vi "CommandZaber.vi"(0 "Zaber":T2={"Serial port handle"="", "Axis"="", "Controller #"=0, "Min position"=0.0, "Max position"=0.0, "Min velocity"=0.0, "Max velocity"=0.0, "Firmware"="", "Device ID"=0, "Variable event"=refnum, "Variable ref"=refnum, "Resolution, usteps/step"=0, "Serial port semaphore"=refnum, "Joystick buttons"={"MinDir"=1, "MaxDir"=2, "MedSpeed"=5, "HighSpeed"=6}} {"Joystick buttons"."HighSpeed" min=1 max=25 step=1; "Joystick buttons"."MedSpeed" min=1 max=25 step=1; "Joystick buttons"."MaxDir" min=1 max=25 step=1; "Joystick buttons"."MinDir" min=1 max=25 step=1}, 2 "Command":T1, 5 "error in":errorcluster) -> (11 "Command time, ms":u32, 14 "Zaber out":T2={"Serial port handle"="", "Axis"="", "Controller #"=0, "Min position"=0.0, "Max position"=0.0, "Min velocity"=0.0, "Max velocity"=0.0, "Firmware"="", "Device ID"=0, "Variable event"=refnum, "Variable ref"=refnum, "Resolution, usteps/step"=0, "Serial port semaphore"=refnum, "Joystick buttons"={"MinDir"=1, "MaxDir"=2, "MedSpeed"=5, "HighSpeed"=6}} {"Joystick buttons"."HighSpeed" min=1 max=25 step=1; "Joystick buttons"."MedSpeed" min=1 max=25 step=1; "Joystick buttons"."MaxDir" min=1 max=25 step=1; "Joystick buttons"."MinDir" min=1 max=25 step=1}, 16 "Answer":T1, 19 "error out":errorcluster)   [LabVIEW 2018]
uses:
  Zaber.ctl
  GenericDataEvent/GenericEvent.ctl
  ZaberVariables.ctl
  CommandZaber.ctl
panel:
  out "Bytes at Port":u32
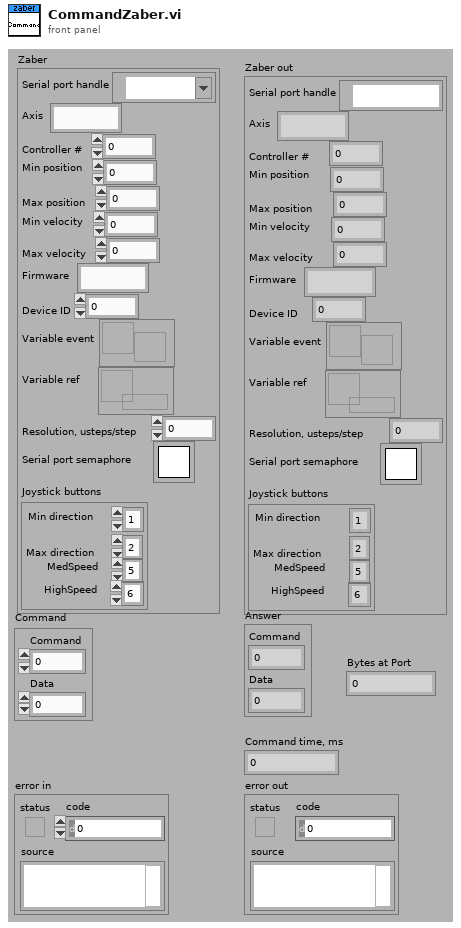
[diagram p1: front panel]
types:
  T1 = typedef "CommandZaber.ctl" = cluster{"Command":u8, "Data":i32}
  T2 = typedef "Zaber.ctl" = cluster{"Serial port handle":refnum<visa-resource-name>, "Axis":string, "Controller #":u8, "Min position":dbl, "Max position":dbl, "Min velocity":dbl, "Max velocity":dbl, "Firmware":string, "Device ID":i32, "Variable event":T3, "Variable ref":refnum<data-value>, "Resolution, usteps/step":i32, "Serial port semaphore":T4, "Joystick buttons":cluster{"MinDir":i32, "MaxDir":i32, "MedSpeed":i32, "HighSpeed":i32}}
  T3 = typedef "GenericEvent.ctl" = refnum<user-event>
  T4 = typedef "Semaphore RefNum" = refnum<k1>
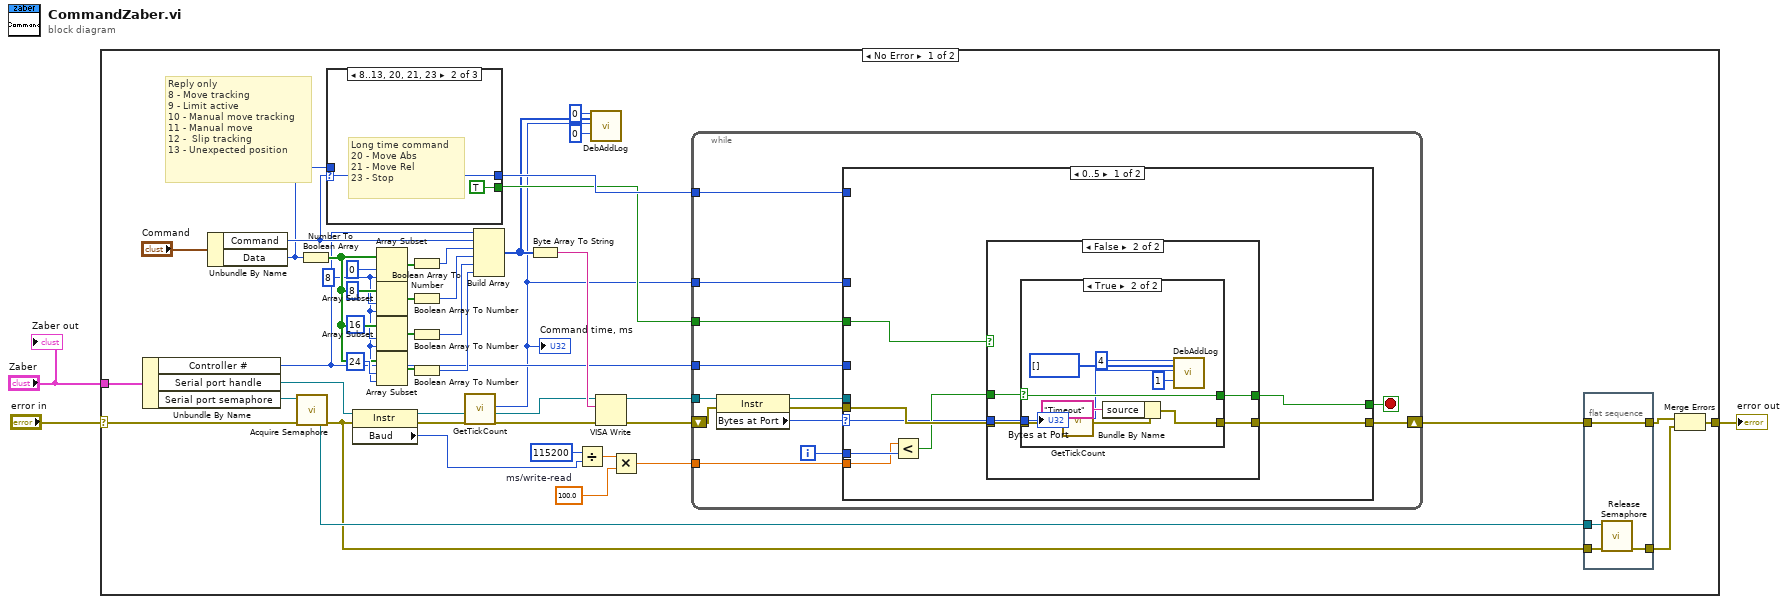
[diagram p0: block diagram]
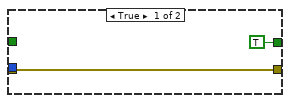
[diagram p2: hidden frame]
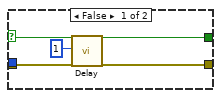
[diagram p3: hidden frame]
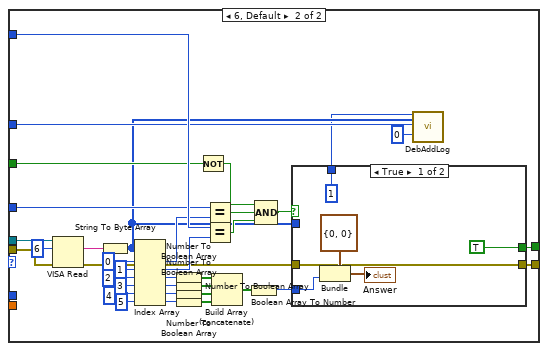
[diagram p4: hidden frame]
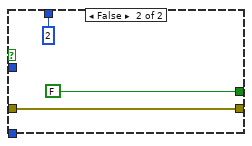
[diagram p5: hidden frame]
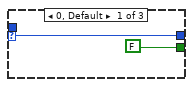
[diagram p6: hidden frame]
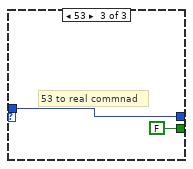
[diagram p7: hidden frame]
diagram:
  n1 = case shown="No Error" "error in" {
    selector: "error in" -> [w26 w145]
    tunnel: [w47 w145] -> w2
    tunnel: "Zaber" -> [w46 _]
    frame No Error {
      w13 = 100.0  # ms/write-read
      w19 = 8 ("length")
      # "Reply only\n8 - Move tracking\n9 - Limit active\n10 - Manual move tracking\n11 - Manual move\n12 -  Slip tracking\n13 - Unexpected position"
      n2 = Unbundle By Name(w46) -> ("Controller #"=w18:u8, "Serial port handle"=w17:refnum<visa-resource-name>, "Serial port semaphore"=w25:T4)
      n3 = Unbundle By Name("Command") -> ("Command"=w28:u8, "Data"=w20:i32)
      n4 = call <vilib>:"Acquire Semaphore.vi"("error in (no error)"=w26, "semaphore"=w25) -> ("error out"=w16:errorcluster, "semaphore out"=w22:T4)  [unwired: 3 in, 1 out]
      n5 = Number To Boolean Array(number=w20) -> (Boolean array=w41:bool[])
      n6 = case shown="8..13, 20, 21, 23" w28 {
        selector: w28 -> [w135 w137 _]
        tunnel: [FALSE TRUE FALSE] -> w8
        tunnel: [w135 w137 w140] -> w21
        tunnel: w20 -> [_ _ w140]
        frame 0, Default {
        }
        frame 8..13, 20, 21, 23 {
          # "Long time command\n20 - Move Abs\n21 - Move Rel\n23 - Stop"
        }
        frame 53 {
          # "53 to real commnad"
        }
      }
      n7 = property class="Instr"(reference=w17, error in=w16) -> (reference out=w9:refnum<visa-resource-name>, error out=w10:errorcluster, "Baud"=w11:u32)
      n8 = Array Subset(array=w41, index=0, length=w19) -> (w33:bool[])
      n9 = Array Subset(array=w41, index=8, length=w19) -> (w38:bool[])
      n10 = Array Subset(array=w41, index=16, length=w19) -> (w40:bool[])
      n11 = Array Subset(array=w41, index=24, length=w19) -> (w43:bool[])
      n12 = Boolean Array To Number(Boolean array=w33) -> (number=w34:u32)
      n13 = Boolean Array To Number(Boolean array=w38) -> (number=w39:u32)
      n14 = Boolean Array To Number(Boolean array=w40) -> (number=w45:u32)
      n15 = Boolean Array To Number(Boolean array=w43) -> (number=w44:u32)
      n16 = call "GetTickCount.vi"("error in (no error)"=w10) -> ("ms"=w5:u32, "error IO"=w27:errorcluster)  [unwired: 17 in]
      "Command time, ms" <- w5
      n17 = Build Array(w18, w28, w34, w39, w45, w44) -> (w6:u32[])
      n18 = Byte Array To String(unsigned byte array=w6) -> (string=w29:string)
      n19 = Divide(x=115200, y=w11) -> (x/y=w14:dbl)
      n20 = call "DebAddLog.vi"("Type"=0, "Log"=w6, "Time"=w5, "Error"=0) -> ()  [unwired: 15 in, 1 out]
      n21 = VISA Write(VISA resource name=w9, write buffer=w29, error in (no error)=w27) -> (VISA resource name out=w32:refnum<visa-resource-name>, error out=w31:errorcluster)  [unwired: 1 out]
      n22 = Multiply(x=w14, y=w13) -> (x*y=w12:dbl)
      n23 = while {
        tunnel: w32 -> [w59]
        tunnel: w21 -> [w57]
        shift-right: [w55] -> w24
        shift-left: w31 -> [w56]
        tunnel: w18 -> [w53]
        tunnel: w12 -> [w52]
        tunnel: w8 -> [w50]
        tunnel: w5 -> [w49]
        i -> [w54]
        stop <- w58 stop-if-true
        n24 = property class="Instr"(reference=w59, error in=w56) -> (reference out=w60:refnum<visa-resource-name>, error out=w61:errorcluster, "Bytes at Port"=w51:u32)
        n25 = case shown="0..5" w51 {
          selector: w51 -> [w62 _]
          tunnel: w60 -> [_ w110]
          tunnel: w61 -> [w67 w109]
          tunnel: [w65 w105] -> w58
          tunnel: w57 -> [_ w104]
          tunnel: [w66 w106] -> w55
          tunnel: w54 -> [w69 _]
          tunnel: w53 -> [_ w103]
          tunnel: w52 -> [w68 _]
          tunnel: w50 -> [w63 w97]
          tunnel: w49 -> [_ w93]
          frame 0..5 {
            n26 = Less?(x=w68, y=w69) -> (x < y?=w64:bool)
            n27 = case shown="False" w63 {
              tunnel: w67 -> [w71 w76]
              tunnel: [w71 w75] -> w66
              tunnel: [TRUE w74] -> w65
              tunnel: w64 -> [_ w73]
              tunnel: w62 -> [_ w72]
              frame True {
              }
              frame False {
                n28 = case shown="True" w73 {
                  selector: w73 -> [w77 w86]
                  tunnel: w76 -> [w79 w89]
                  tunnel: [w78 w88] -> w75
                  tunnel: [w77 w86] -> w74
                  tunnel: w72 -> [_ w81]
                  frame False {
                    n29 = call "Delay.vi"("Delay, ms"=u32 1, "error in"=w79) -> ("error out"=w78:errorcluster)  [unwired: 17 in]
                  }
                  frame True {
                    n30 = call "GetTickCount.vi"() -> ("ms"=w84:u32)  [unwired: 18 in, 1 out]
                    n31 = Bundle By Name(cluster=w89, "source"="Timeout") -> (w88:errorcluster)
                    n32 = call "DebAddLog.vi"("Type"=4, "Log"=i32[] [], "Time"=w84, "Error"=1) -> ()  [unwired: 15 in, 1 out]
                    "Bytes at Port" <- w81
                  }
                }
              }
            }
          }
          frame 6, Default {
            n33 = VISA Read(VISA resource name=w110, byte count=u32 6, error in (no error)=w109) -> (read buffer=w108:string, error out=w94:errorcluster)  [unwired: 2 out]
            n34 = String To Byte Array(string=w108) -> (unsigned byte array=w92:u8[])
            n35 = Index Array(array=w92, index #1=0 ("index"), index #2=1 ("index"), index #3=2 ("index"), index #4=3 ("index"), index #5=4 ("index"), index #6=5 ("index")) -> (element #1=w102:u8, element #2=w101:u8, element #3=w114:u8, element #4=w113:u8, element #5=w112:u8, element #6=w111:u8)
            n36 = Number To Boolean Array(number=w114) -> (Boolean array=w124:bool[])
            n37 = Number To Boolean Array(number=w113) -> (Boolean array=w123:bool[])
            n38 = Number To Boolean Array(number=w112) -> (Boolean array=w122:bool[])
            n39 = Number To Boolean Array(number=w111) -> (Boolean array=w121:bool[])
            n40 = Not(x=w97) -> (.not. x?=w96:bool)
            n41 = Equal?(x=w103, y=w102) -> (x = y?=w100:bool)
            n42 = Equal?(x=w104, y=w101) -> (x = y?=w99:bool)
            n43 = Build Array (concatenate)(w124, w123, w122, w121) -> (w120:bool[])
            n44 = Boolean Array To Number(Boolean array=w120) -> (number=w107:u32)
            n45 = Compound Arithmetic op=AND(w96, w100, w99) -> (w98:bool)
            n46 = case shown="True" w98 {
              tunnel: w107 -> [w129 _]
              tunnel: w94 -> [w127 w134]
              tunnel: [w127 w134] -> w106
              tunnel: [TRUE FALSE] -> w105
              tunnel: w92 -> [_ _]
              tunnel: [1 ("Type") 2 ("Type")] -> w91
              frame True {
                n47 = Bundle(cluster=T1 {"Command"=0, "Data"=0} ("Command 2"), "Data"=w129) -> (→"Answer":T1)  [unwired: 1 in]
              }
              frame False {
              }
            }
            n48 = call "DebAddLog.vi"("Type"=w91, "Log"=w92, "Time"=w93, "Error"=0) -> ()  [unwired: 15 in, 1 out]
          }
        }
      }
      n49 = flat-sequence {
        tunnel: w16 -> [w144]
        tunnel: [w143] -> w48
        tunnel: w24 -> [w142]
        tunnel: [w142] -> w23
        tunnel: w22 -> [w141]
        frame #0 {
          n50 = call <vilib>:"Release Semaphore.vi"("error in (no error)"=w144, "semaphore"=w141) -> ("error out"=w143:errorcluster)  [unwired: 4 in, 1 out]
        }
      }
      n51 = Merge Errors(w23, w48) -> (w47:errorcluster)
    }
    frame Error {
    }
  }
  "error out" <- w2
  "Zaber out" <- "Zaber"
